vi "Remove (-1) From Array.vi"(11 "Input":i32[](array[numeric])) -> (3 "Output":i32[](array[numeric]))   [LabVIEW 2019, in "Zen Analytics.lvlib" / "Zen Analytics.lvclass"]
uses:
  Zen Analytics.lvclass
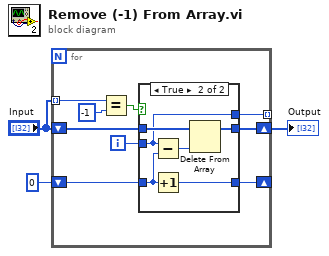
[diagram p0: block diagram]
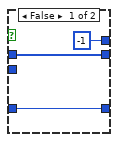
[diagram p2: hidden frame]
diagram:
  n1 = for {
    tunnel: "Input" -> [w7] mode=indexing
    shift-right: [w11] -> _
    shift-left: 0 ("y") -> [w12]
    shift-right: [w8] -> w1
    shift-left: "Input" -> [w9]
    tunnel: [w5] -> _ mode=indexing
    i -> [w10]
    n2 = Equal?(x=w7, y=-1) -> (x = y?=w6:bool)
    n3 = case shown="True" w6 {
      tunnel: w9 -> [w14 w21]
      tunnel: w12 -> [w15 w17]
      tunnel: [w15 w19] -> w11
      tunnel: [w14 w20] -> w8
      tunnel: w10 -> [_ w16]
      tunnel: [-1 w16] -> w5
      frame False {
      }
      frame True {
        n4 = Subtract(x=w16, y=w17) -> (x-y=w18:i32)
        n5 = Increment(x=w17) -> (x+1=w19:i32)
        n6 = Delete From Array(array=w21, index=w18) -> (array with subset deleted=w20:i32[])  [unwired: 1 in, 1 out]
      }
    }
  }
  "Output" <- w1
